vi "Perform Work.vi"(6 "Last request":bool, 8 "error in (no error)":errorcluster, 9 "Initialize":bool, 10 "Reply to":refnum<class "Result Reply Msg.lvclass">, 11 "Pulse Recorder in":refnum<class "Pulse Recorder.lvclass">) -> (0 "error out":errorcluster, 3 "Pulse Recorder out":refnum<class "Pulse Recorder.lvclass">)   [LabVIEW 2016]
uses:
  Pulse Recorder.lvclass
  C:/github/LabActor/Instrument Actor/Instrument Actor.lvclass
  C:/github/LabActor/Worker/Worker.lvclass
  C:/github/LabActor/Template Module/Template Module.lvclass
  C:/Program Files/National Instruments/LabVIEW 2016/vi.lib/ActorFramework/Actor/Actor.lvclass
  Template Module Messages/Result Reply Msg/Result Reply Msg.lvclass
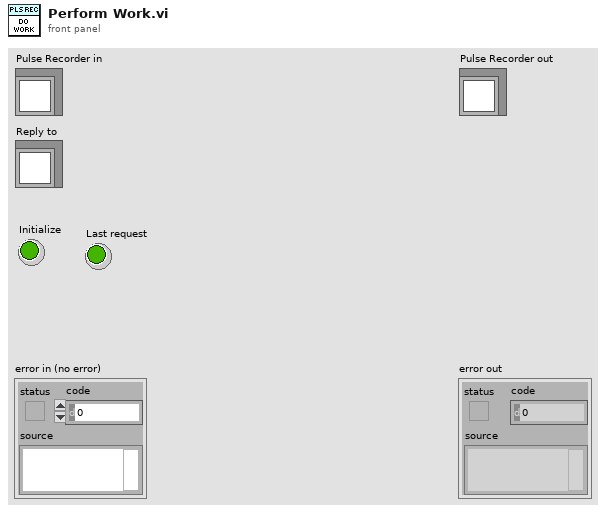
[diagram p1: front panel]
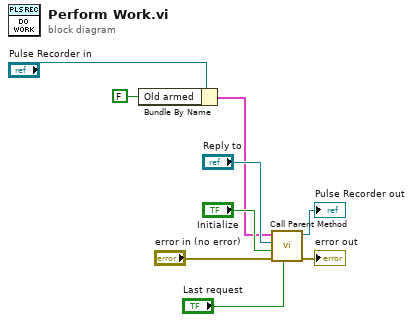
[diagram p0: block diagram]
diagram:
  n1 = Bundle By Name(cluster="Pulse Recorder in", "Old armed"=FALSE ("Armed")) -> (w3:cluster{})
  n2 = call-parent "Call Parent Method"("Last request"="Last request", "error in (no error)"="error in (no error)", "Initialize"="Initialize", "Reply to"="Reply to", "Measure Object in"=w3) -> ("error out"=→"error out":errorcluster, "Measure Object out"=→"Pulse Recorder out":refnum<class "Pulse Recorder.lvclass">)  [unwired: 5 in]
